vi "SetPaneColor.vi"(8 "error in (no error)":errorcluster, 10 "PaneColor":u32(colorbox), 11 "Flex  Dialog (Actor) in":refnum<class "Flex Dialog (Actor).lvclass">) -> (0 "error out":errorcluster, 3 "Flex  Dialog (Actor) out":refnum<class "Flex Dialog (Actor).lvclass">)   [LabVIEW 2014, in "Flex UI Dialog (Actor).lvlib" / "Flex Dialog (Actor).lvclass"]
uses:
  Flex Dialog (Actor).lvclass
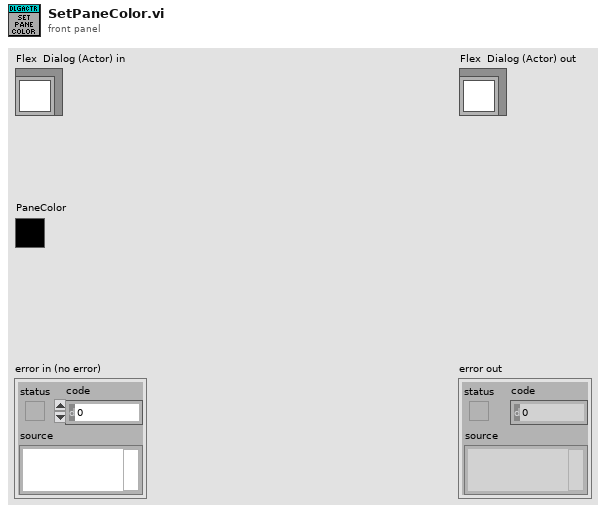
[diagram p1: front panel]
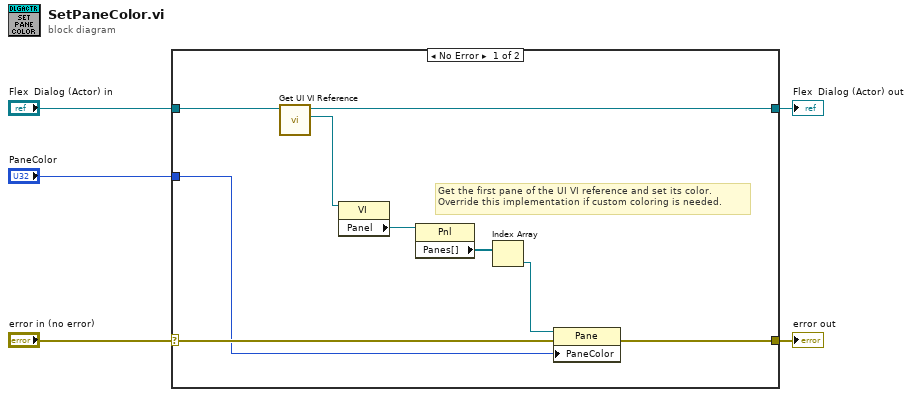
[diagram p0: block diagram]
diagram:
  n1 = case shown="No Error" "error in (no error)" {
    selector: "error in (no error)" -> [w11 w16]
    tunnel: [w10 w16] -> w4
    tunnel: [w8 w15] -> w2
    tunnel: "Flex  Dialog (Actor) in" -> [w7 w15]
    tunnel: "PaneColor" -> [w9 _]
    frame No Error {
      # "Get the first pane of the UI VI reference and set its color.\nOverride this implementation if custom coloring is needed."
      n2 = call-dynamic "Get UI VI Reference.vi"("Flex UI (Actor) in"=w7) -> ("UI VI Reference"=w6:refnum<vi>, "Flex UI (Actor) out"=w8:refnum<class "Flex Dialog (Actor).lvclass">)  [unwired: 8 in, 1 out]
      n3 = property class="VI"(reference=w6) -> ("Panel"=w14:refnum<vi>)  [unwired: 1 in, 2 out]
      n4 = property class="Pnl"(reference=w14) -> ("Panes[]"=w13:refnum<vi>[])  [unwired: 1 in, 2 out]
      n5 = Index Array(array=w13) -> (element=w12:refnum<vi>)  [unwired: 1 in]
      n6 = property class="Pane"(reference=w12, error in=w11, "PaneColor"=w9) -> (error out=w10:errorcluster)  [unwired: 1 out]
    }
    frame Error {
    }
  }
  "error out" <- w4
  "Flex  Dialog (Actor) out" <- w2
